vi "Main Page.vi"(8 "error in (no error)":errorcluster, 11 "Node Ptr":T2 format="%.0x") -> (0 "error out":errorcluster)   [LabVIEW 2019, in "Ghost Bus Addon System Explorer.lvlib"]
uses:
  Ghost Bus Addon System Explorer.lvlib
  <vilib>/NI VeriStand/Custom Device API/Custom Device Item Ref.ctl
  <vilib>/NI/NI VeriStand Hardware Resource Discovery/_Types/Filter Type.ctl
  Addon Shared/SubVIs/GUID Lookup.vi
  <vilib>/NI VeriStand/Custom Device API/NI VeriStand - Get Item Property.vi
  <vilib>/NI VeriStand/Custom Device API/Get Item Property (Boolean).vi
  <vilib>/NI VeriStand/Custom Device API/Get Item Property (String).vi
  <vilib>/NI VeriStand/Custom Device API/Get Item Property (Dependent File).vi
  <vilib>/NI VeriStand/Custom Device API/Custom Device API.lvlib
  <vilib>/NI/NI VeriStand Hardware Resource Discovery/NIVS Hardware Discovery.lvlib
  Addon Shared/Ghost Bus Addon Shared.lvlib
  Addon Shared/Types/986x.ctl
panel:
  in  "Header":cluster{"Section Name":string}={"Section Name"="Addon Settings"}
  in  "Tab Control":T1(tab)
  in  "Primary FD ISO Mode":u32(ring) items=["ISO", "Non ISO", "ISO Legacy"]
  in  "Description":string
  in  "Name":string
  out "Version":string
  in  "Primary Port":string
  in  "Primary CAN Browse":bool
  out "XNET Database":refnum<k21>
  out "XNET Cluster":refnum<k21>
  out "Primary I/O Mode":u32(ring) items=["CAN 2.0", "CAN FD", "CAN FD+BRS"]
  in  "Primary Baud Rate":u64
  in  "Primary Termination":enum16{"Off", "On"}(ring)
  in  "Primary FD Baud Rate":u64
  in  "Primary Loop Priority":i32=100 format="%.0p"
  in  "Ghost FD ISO Mode":u32(ring) items=["ISO", "Non ISO", "ISO Legacy"]
  in  "Ghost Port":string
  in  "Ghost CAN Browse":bool
  in  "Ghost I/O Mode":u32(ring) items=["CAN 2.0", "CAN FD", "CAN FD+BRS"]
  in  "Ghost Baud Rate":u64
  in  "Ghost Termination":enum16{"Off", "On"}(ring)
  in  "Ghost FD Baud Rate":u64
  in  "Ghost Loop Priority":i32=100 format="%.0p"
  in  "RIO Device":string
  in  "Bitfile Path":path
  in  "Enable Bitfile":bool
  in  "RIO Browse":bool
  in  "SHDocVw.IWebBrowser2":refnum<k7>(container)
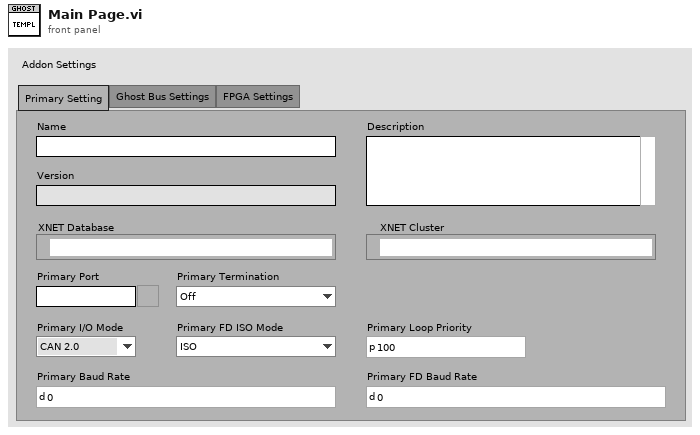
[diagram p1: front panel]
types:
  T1 = enum32{"Primary Setting", "Ghost Bus Settings", "FPGA Settings"}
  T2 = typedef "Custom Device API.lvlib/Custom Device Item Ref.ctl" = u64
  T3 = typedef "Ghost Bus Addon Shared.lvlib/XNET Settings.ctl" = cluster{"Database":refnum<k21>, "Cluster":refnum<k21>, "Primary":T4, "Ghost":T4}
  T4 = typedef "Ghost Bus Addon Shared.lvlib/XNET Port Settings.ctl" = cluster{"Port":string, "Baud Rate":u64, "Termination":u32, "CAN I/O Mode":u32, "FD Baud Rate":u64, "Priority":i32, "FD ISO Mode":u32}
  T5 = typedef "Custom Device API.lvlib/Custom Device Item Info.ctl" = cluster{"Name":string, "Is Channel":bool, "GUID":string, "Is Waveform":bool}
  T6 = typedef "986x.ctl" = cluster{"Enable":bool, "RIO Device":string, "Bitfile":path}
  T7 = typedef "NIVS Hardware Discovery.lvlib/Filter Type.ctl" = enum16{"Device Category", "Product Name", "Ethernet", "XNET", "VISA", "FPGA", "EtherCAT Master", "DAQmx", "GPIB", "Serial"}
  T8 = typedef "Custom Device API.lvlib/Custom Device Commands.ctl" = enum16{"Default", "Item renamed", "Shutdown", "Dynamic button pressed"}
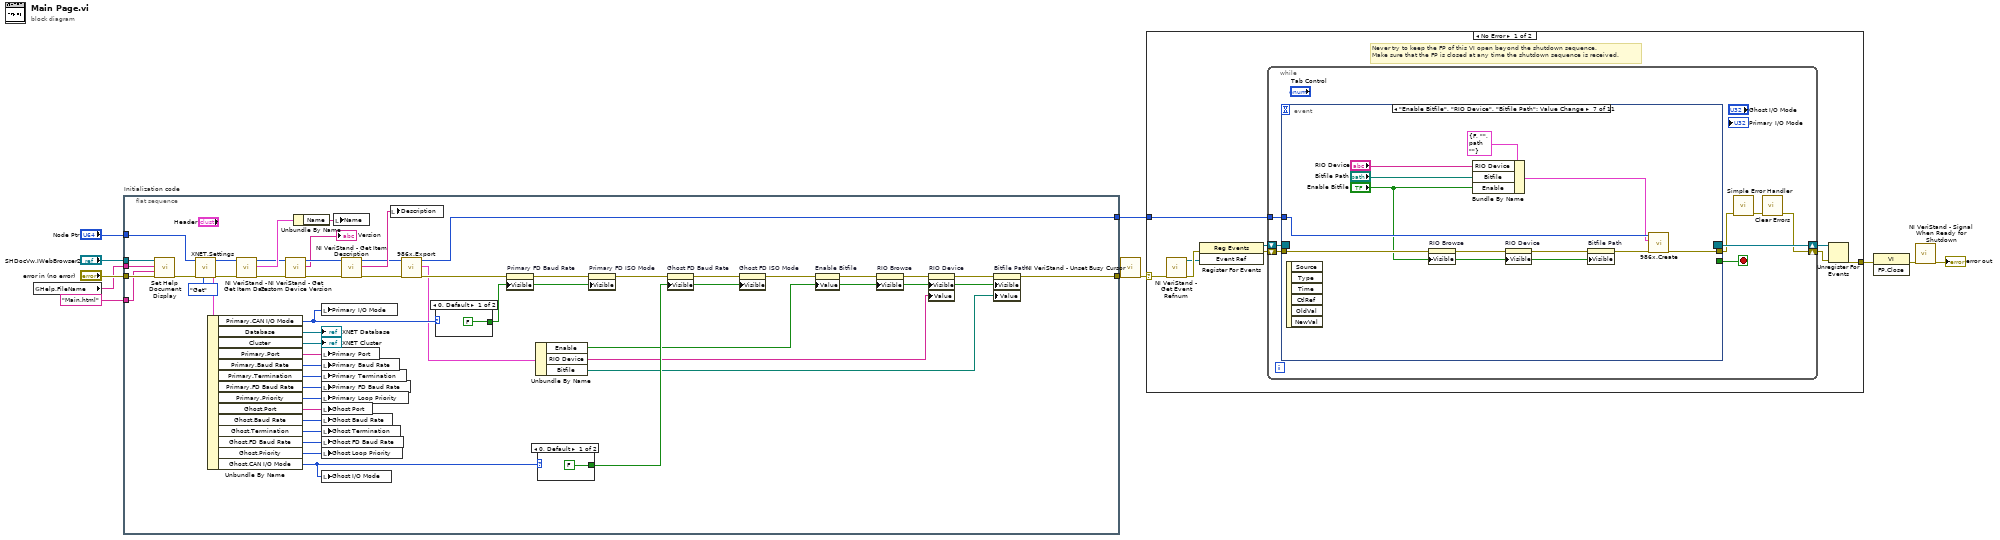
[diagram p0: block diagram]
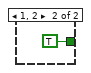
[diagram p2: hidden frame]
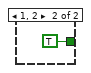
[diagram p3: hidden frame]
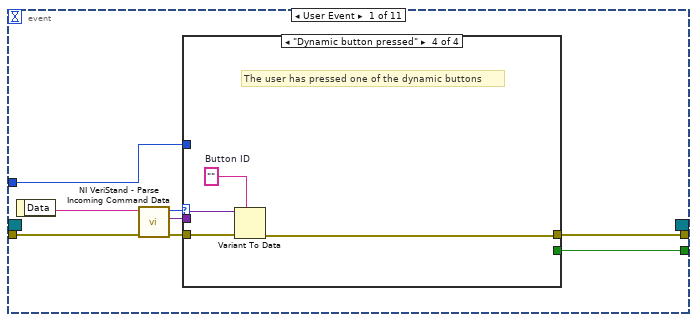
[diagram p4: hidden frame]
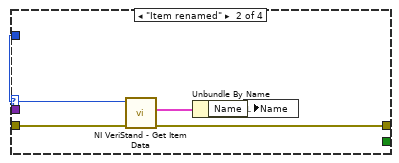
[diagram p6: hidden frame]
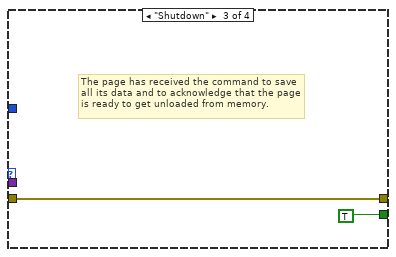
[diagram p7: hidden frame]
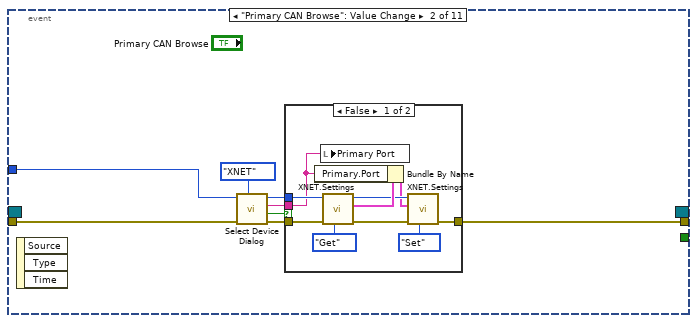
[diagram p8: hidden frame]
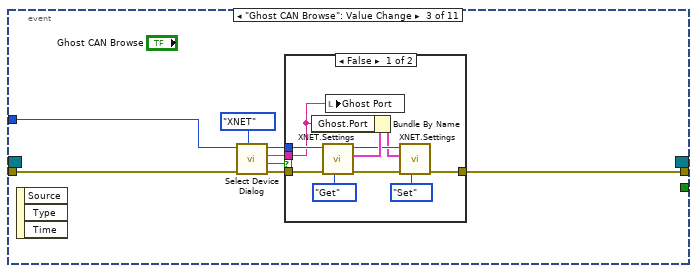
[diagram p10: hidden frame]
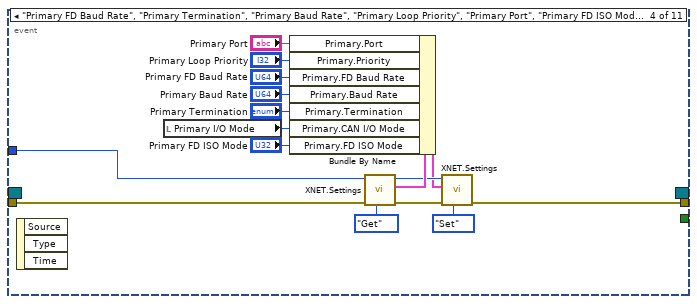
[diagram p12: hidden frame]
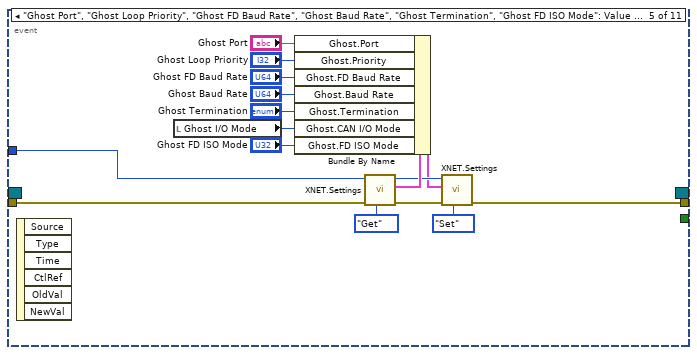
[diagram p13: hidden frame]
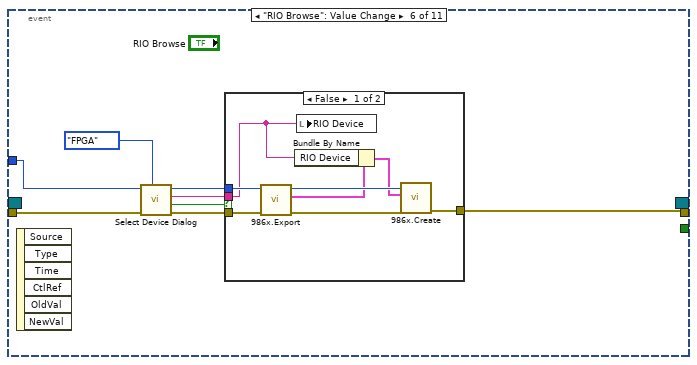
[diagram p14: hidden frame]
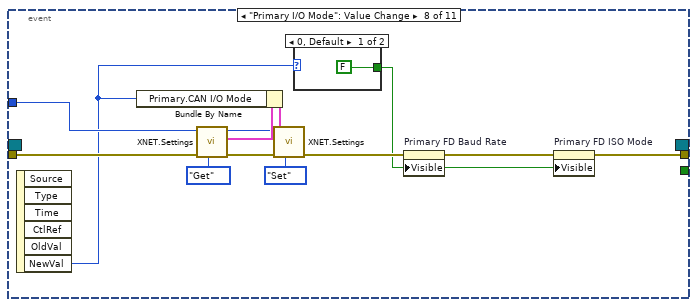
[diagram p16: hidden frame]
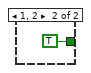
[diagram p17: hidden frame]
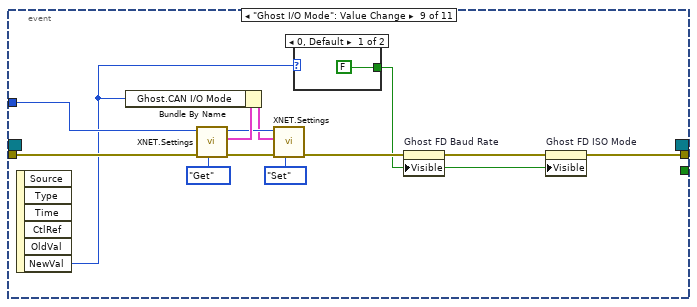
[diagram p18: hidden frame]
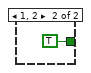
[diagram p19: hidden frame]
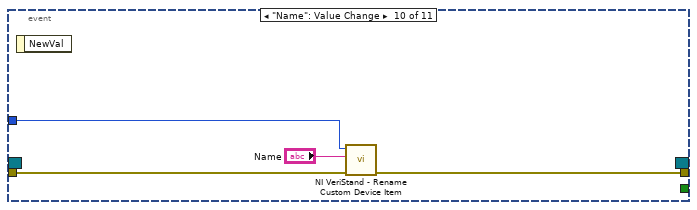
[diagram p20: hidden frame]
diagram:
  n1 = global read "GUID Lookup.vi" "Help.FileName"() -> (w1:string)
  n2 = flat-sequence "Initialization code" {
    tunnel: "error in (no error)" -> [w59]
    tunnel: "Node Ptr" -> [w36]
    tunnel: [w15] -> w7
    tunnel: [w21] -> w4
    tunnel: "SHDocVw.IWebBrowser2" -> [w58]
    tunnel: w1 -> [w57]
    tunnel: "Main.html" ("HTML File") -> [w56]
    frame #0 {
      n3 = call "Set Help Document Display.vi"("error in (no error)"=w59, "HTML File"=w56, "Main CHM File"=w57, "SHDocVw.IWebBrowser2"=w58) -> ("error out"=w37:errorcluster)  [unwired: 7 in]
      n4 = call "XNET.Settings.vi"("Action"=enum8{"Get", "Set"}."Get", "error in (no error)"=w37, "Parent Ref in"=w36) -> ("error out"=w55:errorcluster, "XNET Settings"=w52:T3, "Item Ref out"=w54:T2)  [unwired: 6 in]
      n5 = Unbundle By Name(w52) -> ("Primary.CAN I/O Mode"=w44:u32, "Database"=→"XNET Database":refnum<k21>, "Cluster"=→"XNET Cluster":refnum<k21>, "Primary.Port"=w49:string, "Primary.Baud Rate"=w48:u64, "Primary.Termination"=w47:u32, "Primary.FD Baud Rate"=w46:u64, "Primary.Priority"=w45:i32, "Ghost.Port"=w32:string, "Ghost.Baud Rate"=w31:u64, "Ghost.Termination"=w30:u32, "Ghost.FD Baud Rate"=w29:u64, "Ghost.Priority"=w33:i32, "Ghost.CAN I/O Mode"=w25:u32)
      n6 = call <vilib>:"NI VeriStand - Get Item Data.vi"("error in (no error)"=w55, "Item Ref in"=w54) -> ("error out"=w43:errorcluster, "Item Info"=w61:T5, "Item Ref out"=w42:T2)  [unwired: 7 out]
      n7 = call <vilib>:"NI VeriStand - Get Custom Device Version.vi"("error in (no error)"=w43, "Device Ref in"=w42) -> ("error out"=w39:errorcluster, "Value"=→"Version":string, "Device Ref out"=w41:T2)  [unwired: 7 in]
      n8 = Unbundle By Name(w61) -> ("Name"=w60:string)
      n9 = local write "Primary I/O Mode"(w44) -> ()
      n10 = local write "Primary Port"(w49) -> ()
      n11 = local write "Primary Baud Rate"(w48) -> ()
      n12 = local write "Primary Termination"(w47) -> ()
      n13 = local write "Primary FD Baud Rate"(w46) -> ()
      n14 = local write "Primary Loop Priority"(w45) -> ()
      n15 = local write "Ghost Port"(w32) -> ()
      n16 = local write "Ghost Baud Rate"(w31) -> ()
      n17 = local write "Ghost Termination"(w30) -> ()
      n18 = local write "Ghost FD Baud Rate"(w29) -> ()
      n19 = local write "Ghost Loop Priority"(w33) -> ()
      n20 = local write "Ghost I/O Mode"(w25) -> ()
      n21 = local write "Name"(w60) -> ()
      n22 = call <vilib>:"NI VeriStand - Get Item Description.vi"("error in (no error)"=w39, "Item Ref in"=w41) -> ("error out"=w24:errorcluster, "Description"=w38:string, "Item Ref out"=w22:T2)  [unwired: 6 in, 1 out]
      n23 = local write "Description"(w38) -> ()
      n24 = call "986x.Export.vi"("error in (no error)"=w24, "Device Item Ref in"=w22) -> ("error out"=w23:errorcluster, "986x Support"=w20:T6, "Item Ref out"=w21:T2)  [unwired: 7 in]
      n25 = case shown="0, Default" w44 {
        tunnel: [FALSE TRUE] -> w34
        frame 0, Default {
        }
        frame 1, 2 {
        }
      }
      n26 = property on="Primary FD Baud Rate" class="DigNum (strict)"(error in=w23, "Visible"=w34) -> (error out=w35:errorcluster)  [unwired: 1 in, 1 out]
      n27 = Unbundle By Name(w20) -> ("Enable"=w14:bool, "RIO Device"=w13:string, "Bitfile"=w12:path)
      n28 = case shown="0, Default" w25 {
        tunnel: [FALSE TRUE] -> w28
        frame 0, Default {
        }
        frame 1, 2 {
        }
      }
      n29 = property on="Primary FD ISO Mode" class="Ring (strict)"(error in=w35, "Visible"=w34) -> (error out=w26:errorcluster)  [unwired: 1 in, 1 out]
      n30 = property on="Ghost FD Baud Rate" class="DigNum (strict)"(error in=w26, "Visible"=w28) -> (error out=w27:errorcluster)  [unwired: 1 in, 1 out]
      n31 = property on="Ghost FD ISO Mode" class="Ring (strict)"(error in=w27, "Visible"=w28) -> (error out=w19:errorcluster)  [unwired: 1 in, 1 out]
      n32 = property on="Enable Bitfile" class="Bool (strict)"(error in=w19, "Value"=w14) -> (error out=w18:errorcluster)  [unwired: 1 in, 1 out]
      n33 = property on="RIO Browse" class="Bool"(error in=w18, "Visible"=w14) -> (error out=w17:errorcluster)  [unwired: 1 in, 1 out]
      n34 = property on="RIO Device" class="Str"(error in=w17, "Visible"=w14, "Value"=w13) -> (error out=w16:errorcluster)  [unwired: 1 in, 1 out]
      n35 = property on="Bitfile Path" class="Path"(error in=w16, "Visible"=w14, "Value"=w12) -> (error out=w15:errorcluster)  [unwired: 1 in, 1 out]
    }
  }
  n36 = call <vilib>:"NI VeriStand - Unset Busy Cursor.vi"("error in (no error)"=w7) -> ("error out"=w6:errorcluster)  [unwired: 10 out]
  n37 = case shown="No Error" w6 {
    selector: w6 -> [w66 w241]
    tunnel: [w71 w239] -> w11
    tunnel: w4 -> [w67 _]
    frame No Error {
      # "Never try to keep the FP of this VI open beyond the shutdown sequence.\nMake sure that the FP is closed at any time the shutdown sequence is received."
      n38 = call <vilib>:"NI VeriStand - Get Event Refnum.vi"("error in (no error)"=w66) -> ("error out"=w74:errorcluster, "Event Ref"=w70:refnum<user-event>)  [unwired: 9 out]
      n39 = register-events(error in=w74, w70) -> (reference out=w68:refnum<event-registration>, error out=w69:errorcluster)  [unwired: 1 in]
      n40 = while {
        tunnel: w67 -> [w78]
        shift-right: [w75] -> w72
        shift-left: w69 -> [w81]
        shift-right: [w82] -> w73
        shift-left: w68 -> [w80]
        stop <- w79 stop-if-true
        n41 = event shown="[6] \"Enable Bitfile\", \"RIO Device\", \"Bitfile Path\": Value Change" {
          selector: w80 -> [_ _ _ _ _ _ _ _ _ _ _]
          dyn-events: [_ _ _ _ _ _ _ _ _ _ _] -> w82
          timeout: _ -> [_ _ _ _ _ _ _ _ _ _ _]
          tunnel: w81 -> [w90 w105 w124 w150 w166 w178 w198 w207 w222 w234 w238]
          tunnel: [w86 _ _ _ _ _ _ _ _ _ _] -> w79
          tunnel: [w85 w103 w122 w149 w165 w173 w199 w202 w217 w233 w237] -> w77
          tunnel: w78 -> [w84 w104 w123 w148 w164 w179 w200 w206 w221 w232 w236]
          event User Event {
            n42 = event-data() -> ("Data"=w89:string)  [unwired: 1 out]
            n43 = call <vilib>:"NI VeriStand - Parse Incoming Command Data.vi"("error in (no error)"=w90, "Incoming data"=w89) -> ("error out"=w88:errorcluster, "Outgoing data"=w83:variant, "Action"=w87:T8)  [unwired: 7 out]
            n44 = case shown="\"Dynamic button pressed\"" w87 {
              tunnel: w88 -> [w91 w96 w97 w102]
              tunnel: [_ _ TRUE _] -> w86
              tunnel: [w91 w93 w97 w99] -> w85
              tunnel: w84 -> [_ w95 _ _]
              tunnel: w83 -> [_ _ _ w101]
              frame "Default", Default {
              }
              frame "Item renamed" {
                n45 = call <vilib>:"NI VeriStand - Get Item Data.vi"("error in (no error)"=w96, "Item Ref in"=w95) -> ("error out"=w93:errorcluster, "Item Info"=w94:T5)  [unwired: 8 out]
                n46 = Unbundle By Name(w94) -> ("Name"=w92:string)
                n47 = local write "Name"(w92) -> ()
              }
              frame "Shutdown" {
                # "The page has received the command to save all its data and to acknowledge that the page is ready to get unloaded from memory."
              }
              frame "Dynamic button pressed" {
                w100 = ""  # Button ID
                # "The user has pressed one of the dynamic buttons"
                n48 = Variant To Data(error in=w102, type=w100, Variant=w101) -> (error out=w99:errorcluster)  [unwired: 1 out]
              }
            }
          }
          event "Primary CAN Browse": Value Change {
            n49 = event-data() -> ()  [unwired: 4 out]
            n50 = call <vilib>:"Select Device Dialog.vi"("Filter Type"=Filter_Type."XNET", "error in (no error)"=w105, "Item Ref in"=w104) -> ("error out"=w109:errorcluster, "Cancelled?"=w108:bool, "Selected Alias"=w107:string, "Item Ref out"=w110:T2)  [unwired: 5 in]
            n51 = case shown="False" w108 {
              tunnel: w110 -> [w118 _]
              tunnel: [w115 w121] -> w103
              tunnel: w109 -> [w112 w121]
              tunnel: w107 -> [w111 _]
              frame False {
                n52 = local write "Primary Port"(w111) -> ()
                n53 = call "XNET.Settings.vi"("Action"=enum8{"Get", "Set"}."Get", "error in (no error)"=w112, "Parent Ref in"=w118) -> ("error out"=w113:errorcluster, "XNET Settings"=w119:T3, "Item Ref out"=w116:T2)  [unwired: 6 in]
                n54 = Bundle By Name(cluster=w119, "Primary.Port"=w111) -> (w114:T3)
                n55 = call "XNET.Settings.vi"("Action"=enum8{"Get", "Set"}."Set", "error in (no error)"=w113, "XNET Settings"=w114, "Parent Ref in"=w116) -> ("error out"=w115:errorcluster)  [unwired: 5 in, 2 out]
              }
              frame True {
              }
            }
          }
          event "Ghost CAN Browse": Value Change {
            n56 = event-data() -> ()  [unwired: 4 out]
            n57 = call <vilib>:"Select Device Dialog.vi"("Filter Type"=Filter_Type."XNET", "error in (no error)"=w124, "Item Ref in"=w123) -> ("error out"=w128:errorcluster, "Cancelled?"=w127:bool, "Selected Alias"=w126:string, "Item Ref out"=w129:T2)  [unwired: 5 in]
            n58 = case shown="False" w127 {
              tunnel: w129 -> [w137 _]
              tunnel: [w134 w140] -> w122
              tunnel: w128 -> [w131 w140]
              tunnel: w126 -> [w130 _]
              frame False {
                n59 = call "XNET.Settings.vi"("Action"=enum8{"Get", "Set"}."Get", "error in (no error)"=w131, "Parent Ref in"=w137) -> ("error out"=w132:errorcluster, "XNET Settings"=w138:T3, "Item Ref out"=w135:T2)  [unwired: 6 in]
                n60 = Bundle By Name(cluster=w138, "Ghost.Port"=w130) -> (w133:T3)
                n61 = local write "Ghost Port"(w130) -> ()
                n62 = call "XNET.Settings.vi"("Action"=enum8{"Get", "Set"}."Set", "error in (no error)"=w132, "XNET Settings"=w133, "Parent Ref in"=w135) -> ("error out"=w134:errorcluster)  [unwired: 5 in, 2 out]
              }
              frame True {
              }
            }
          }
          event "Primary FD Baud Rate", "Primary Termination", "Primary Baud Rate", "Primary Loop Priority", "Primary Port", "Primary FD ISO Mode": Value Change {
            n63 = event-data() -> ()  [unwired: 4 out]
            n64 = local read "Primary I/O Mode"() -> (w142:u32)
            n65 = call "XNET.Settings.vi"("Action"=enum8{"Get", "Set"}."Get", "error in (no error)"=w150, "Parent Ref in"=w148) -> ("error out"=w151:errorcluster, "XNET Settings"=w155:T3, "Item Ref out"=w153:T2)  [unwired: 6 in]
            n66 = Bundle By Name(cluster=w155, "Primary.Port"="Primary Port", "Primary.Priority"="Primary Loop Priority", "Primary.FD Baud Rate"="Primary FD Baud Rate", "Primary.Baud Rate"="Primary Baud Rate", "Primary.Termination"="Primary Termination", "Primary.CAN I/O Mode"=w142, "Primary.FD ISO Mode"="Primary FD ISO Mode") -> (w152:T3)
            n67 = call "XNET.Settings.vi"("Action"=enum8{"Get", "Set"}."Set", "error in (no error)"=w151, "XNET Settings"=w152, "Parent Ref in"=w153) -> ("error out"=w149:errorcluster)  [unwired: 5 in, 2 out]
          }
          event "Ghost Port", "Ghost Loop Priority", "Ghost FD Baud Rate", "Ghost Baud Rate", "Ghost Termination", "Ghost FD ISO Mode": Value Change {
            n68 = event-data() -> ()  [unwired: 7 out]
            n69 = local read "Ghost I/O Mode"() -> (w163:u32)
            n70 = call "XNET.Settings.vi"("Action"=enum8{"Get", "Set"}."Get", "error in (no error)"=w166, "Parent Ref in"=w164) -> ("error out"=w167:errorcluster, "XNET Settings"=w171:T3, "Item Ref out"=w169:T2)  [unwired: 6 in]
            n71 = Bundle By Name(cluster=w171, "Ghost.Port"="Ghost Port", "Ghost.Priority"="Ghost Loop Priority", "Ghost.FD Baud Rate"="Ghost FD Baud Rate", "Ghost.Baud Rate"="Ghost Baud Rate", "Ghost.Termination"="Ghost Termination", "Ghost.CAN I/O Mode"=w163, "Ghost.FD ISO Mode"="Ghost FD ISO Mode") -> (w168:T3)
            n72 = call "XNET.Settings.vi"("Action"=enum8{"Get", "Set"}."Set", "error in (no error)"=w167, "XNET Settings"=w168, "Parent Ref in"=w169) -> ("error out"=w165:errorcluster)  [unwired: 5 in, 2 out]
          }
          event "RIO Browse": Value Change {
            n73 = event-data() -> ()  [unwired: 7 out]
            n74 = call <vilib>:"Select Device Dialog.vi"("Filter Type"=Filter_Type."FPGA", "error in (no error)"=w178, "Item Ref in"=w179) -> ("error out"=w176:errorcluster, "Cancelled?"=w177:bool, "Selected Alias"=w174:string, "Item Ref out"=w175:T2)  [unwired: 5 in]
            n75 = case shown="False" w177 {
              tunnel: w176 -> [w187 w189]
              tunnel: w175 -> [w188 _]
              tunnel: w174 -> [w183 _]
              tunnel: [w184 w189] -> w173
              frame False {
                n76 = call "986x.Export.vi"("error in (no error)"=w187, "Device Item Ref in"=w188) -> ("error out"=w186:errorcluster, "986x Support"=w182:T6, "Item Ref out"=w185:T2)  [unwired: 7 in]
                n77 = Bundle By Name(cluster=w182, "RIO Device"=w183) -> (w181:T6)
                n78 = local write "RIO Device"(w183) -> ()
                n79 = call "986x.Create.vi"("error in (no error)"=w186, "986x Support"=w181, "Device Item Ref in"=w185) -> ("error out"=w184:errorcluster)  [unwired: 7 in, 1 out]
              }
              frame True {
              }
            }
          }
          event "Enable Bitfile", "RIO Device", "Bitfile Path": Value Change {
            n80 = event-data() -> ()  [unwired: 7 out]
            n81 = property on="RIO Browse" class="Bool"(error in=w198, "Visible"="Enable Bitfile") -> (error out=w197:errorcluster)  [unwired: 1 in, 1 out]
            n82 = Bundle By Name(cluster=T6 {"Enable"=FALSE, "RIO Device"="", "Bitfile"=path ""} ("986x Support"), "RIO Device"="RIO Device", "Bitfile"="Bitfile Path", "Enable"="Enable Bitfile") -> (w190:T6)
            n83 = property on="RIO Device" class="Str"(error in=w197, "Visible"="Enable Bitfile") -> (error out=w196:errorcluster)  [unwired: 1 in, 1 out]
            n84 = property on="Bitfile Path" class="Path"(error in=w196, "Visible"="Enable Bitfile") -> (error out=w195:errorcluster)  [unwired: 1 in, 1 out]
            n85 = call "986x.Create.vi"("error in (no error)"=w195, "986x Support"=w190, "Device Item Ref in"=w200) -> ("error out"=w199:errorcluster)  [unwired: 7 in, 1 out]
          }
          event "Primary I/O Mode": Value Change {
            n86 = event-data() -> ("NewVal"=w204:u32)  [unwired: 6 out]
            n87 = call "XNET.Settings.vi"("Action"=enum8{"Get", "Set"}."Get", "error in (no error)"=w207, "Parent Ref in"=w206) -> ("error out"=w208:errorcluster, "XNET Settings"=w212:T3, "Item Ref out"=w210:T2)  [unwired: 6 in]
            n88 = Bundle By Name(cluster=w212, "Primary.CAN I/O Mode"=w204) -> (w209:T3)
            n89 = call "XNET.Settings.vi"("Action"=enum8{"Get", "Set"}."Set", "error in (no error)"=w208, "XNET Settings"=w209, "Parent Ref in"=w210) -> ("error out"=w205:errorcluster)  [unwired: 5 in, 2 out]
            n90 = case shown="0, Default" w204 {
              tunnel: [FALSE TRUE] -> w201
              frame 0, Default {
              }
              frame 1, 2 {
              }
            }
            n91 = property on="Primary FD Baud Rate" class="DigNum (strict)"(error in=w205, "Visible"=w201) -> (error out=w203:errorcluster)  [unwired: 1 in, 1 out]
            n92 = property on="Primary FD ISO Mode" class="Ring (strict)"(error in=w203, "Visible"=w201) -> (error out=w202:errorcluster)  [unwired: 1 in, 1 out]
          }
          event "Ghost I/O Mode": Value Change {
            n93 = event-data() -> ("NewVal"=w219:u32)  [unwired: 6 out]
            n94 = call "XNET.Settings.vi"("Action"=enum8{"Get", "Set"}."Get", "error in (no error)"=w222, "Parent Ref in"=w221) -> ("error out"=w223:errorcluster, "XNET Settings"=w227:T3, "Item Ref out"=w225:T2)  [unwired: 6 in]
            n95 = Bundle By Name(cluster=w227, "Ghost.CAN I/O Mode"=w219) -> (w224:T3)
            n96 = call "XNET.Settings.vi"("Action"=enum8{"Get", "Set"}."Set", "error in (no error)"=w223, "XNET Settings"=w224, "Parent Ref in"=w225) -> ("error out"=w220:errorcluster)  [unwired: 5 in, 2 out]
            n97 = case shown="0, Default" w219 {
              tunnel: [FALSE TRUE] -> w216
              frame 0, Default {
              }
              frame 1, 2 {
              }
            }
            n98 = property on="Ghost FD Baud Rate" class="DigNum (strict)"(error in=w220, "Visible"=w216) -> (error out=w218:errorcluster)  [unwired: 1 in, 1 out]
            n99 = property on="Ghost FD ISO Mode" class="Ring (strict)"(error in=w218, "Visible"=w216) -> (error out=w217:errorcluster)  [unwired: 1 in, 1 out]
          }
          event "Name": Value Change {
            n100 = event-data() -> ()  [unwired: 2 out]
            n101 = call <vilib>:"NI VeriStand - Rename Custom Device Item.vi"("error in (no error)"=w234, "New Name"="Name", "Item Ref in"=w232) -> ("error out"=w233:errorcluster)  [unwired: 1 in, 7 out]
          }
          event "Description": Value Change {
            n102 = event-data() -> ()  [unwired: 2 out]
            n103 = call <vilib>:"NI VeriStand - Set Item Description.vi"("error in (no error)"=w238, "Description"="Description", "Item Ref in"=w236) -> ("error out"=w237:errorcluster)  [unwired: 6 in, 2 out]
          }
        }
        n104 = call <vilib>:"Simple Error Handler.vi"("error in (no error)"=w77) -> ("error out"=w76:errorcluster)  [unwired: 1 in, 7 out]
        n105 = call <vilib>:"Clear Errors.vi"("error in (no error)"=w76) -> ("error out"=w75:errorcluster)  [unwired: 1 in, 5 out]
      }
      n106 = Unregister For Events(event registration refnum=w73, error in=w72) -> (error out=w71:errorcluster)
    }
    frame Error {
      n107 = call <vilib>:"Simple Error Handler.vi"("error in (no error)"=w241) -> ("error out"=w240:errorcluster)  [unwired: 1 in, 7 out]
      n108 = call <vilib>:"Clear Errors.vi"("error in (no error)"=w240) -> ("error out"=w239:errorcluster)  [unwired: 1 in, 5 out]
    }
  }
  n109 = invoke class="VI" method="FP.Close"(error in=w11) -> (error out=w10:errorcluster)  [unwired: 2 in, 2 out]
  n110 = call <vilib>:"NI VeriStand - Signal When Ready for Shutdown.vi"("error in (no error)"=w10) -> ("error out"=→"error out":errorcluster)  [unwired: 10 out]
